vi "Game of colours.vi"() -> ()   [LabVIEW 2018]
uses:
  TypeDefs/State.ctl
  TypeDefs/Application Data.ctl
panel:
  in  "Type the sequence shown":T1
  out "Score":i32
  out "sequence to memorize":u32(colorbox) caption="Sequence to memorize"
  # "The game of colours"
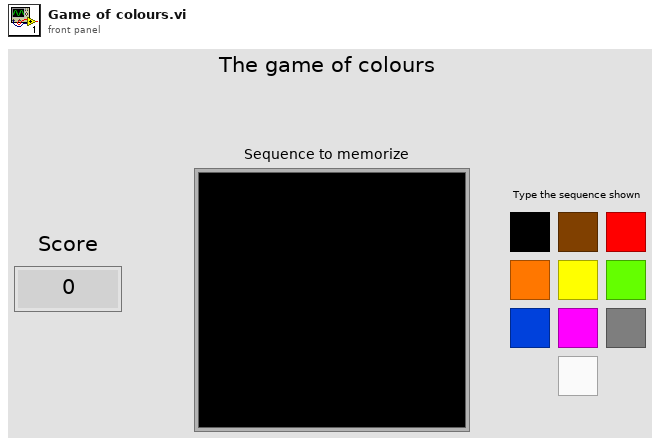
[diagram p1: front panel]
types:
  T1 = cluster{"0":bool, "7":bool, "8":bool, "9":bool, "4":bool, "5":bool, "6":bool, "1":bool, "2":bool, "3":bool}
  T2 = typedef "Application Data.ctl" = cluster{"Sequence":i32[], "Available Colours":u32[], "Wait Time(ms)":u32, "No. Keys Pressed":i32, "Last Key":i16, "Tally":i32}
  T3 = typedef "State.ctl" = enum16{"Initialize", "Add New Colour", "Show Sequence", "Wait for Event", "Check Key Press", "Success", "Failure", "Exit"}
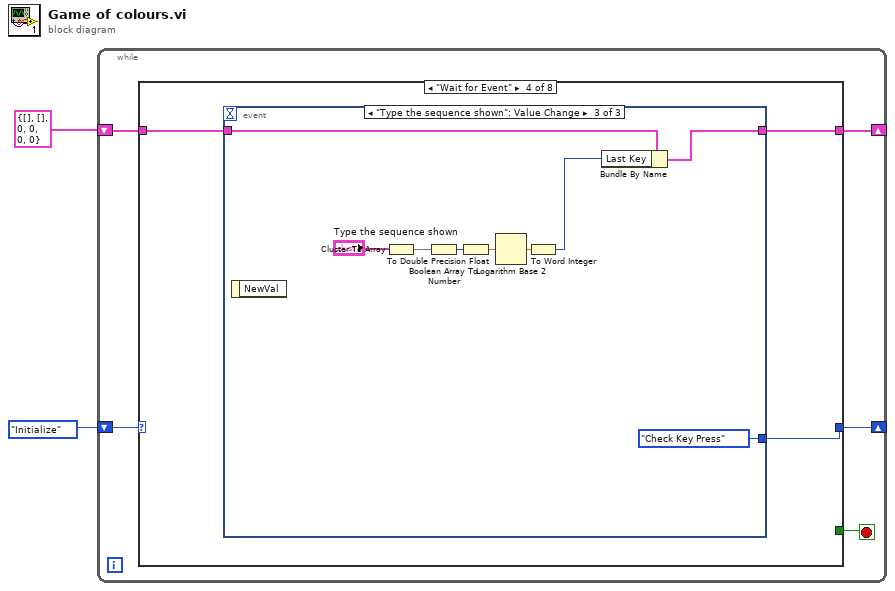
[diagram p0: block diagram]
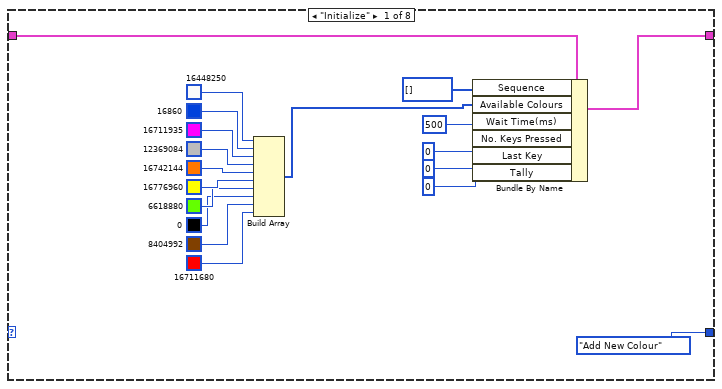
[diagram p2: hidden frame]
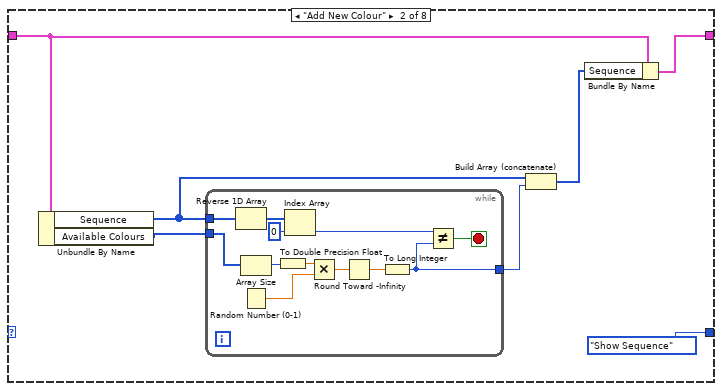
[diagram p3: hidden frame]
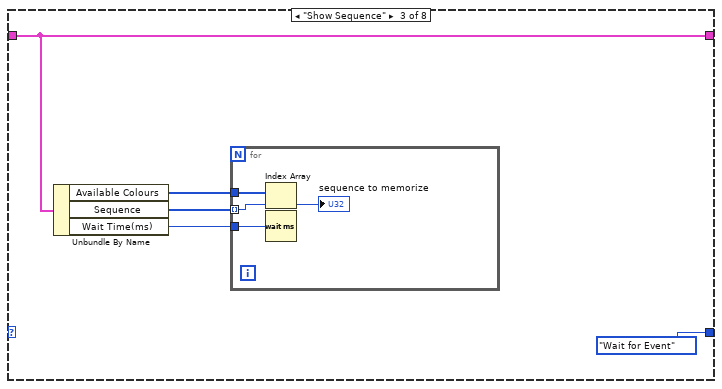
[diagram p4: hidden frame]
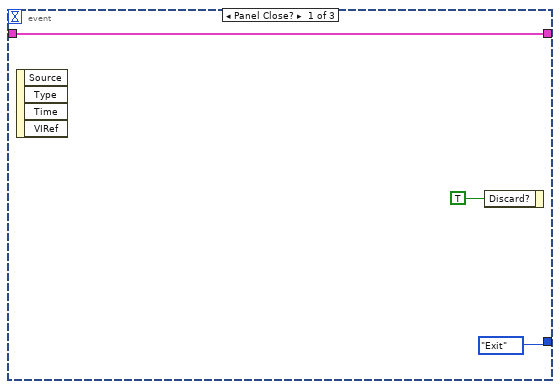
[diagram p5: hidden frame]
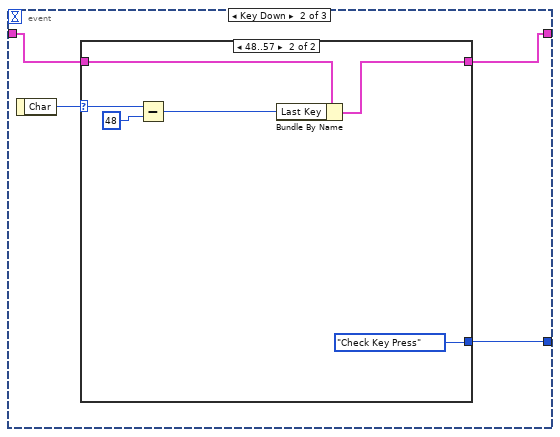
[diagram p6: hidden frame]
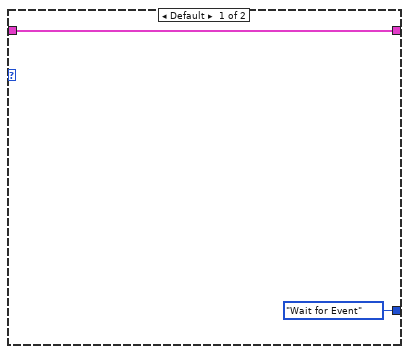
[diagram p7: hidden frame]
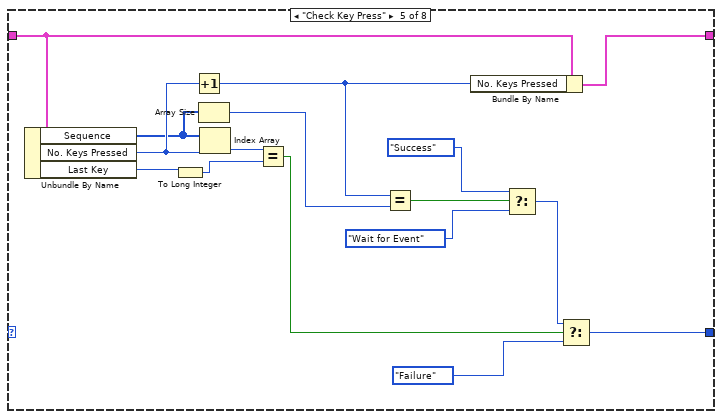
[diagram p8: hidden frame]
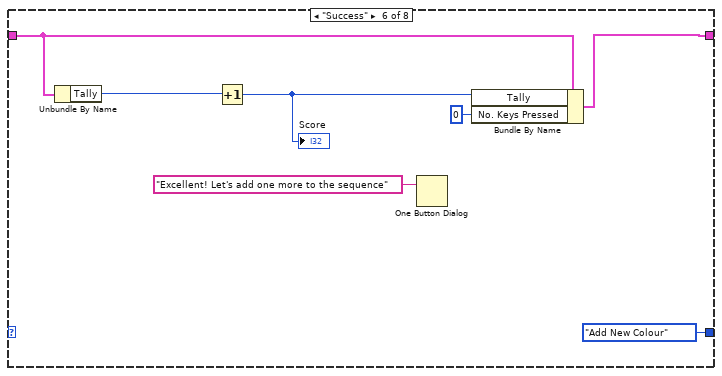
[diagram p9: hidden frame]
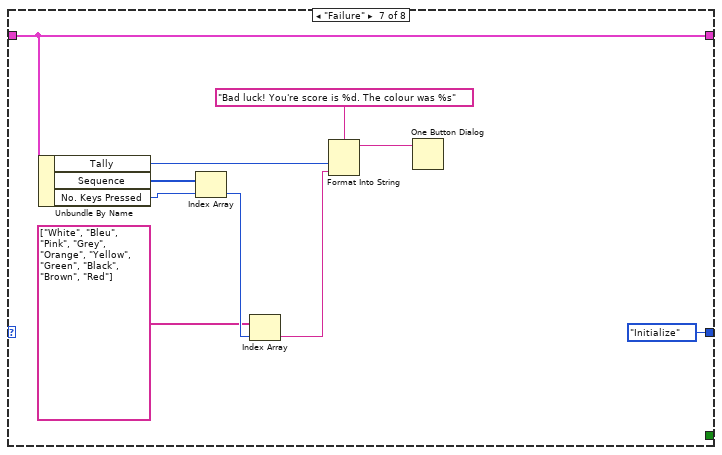
[diagram p10: hidden frame]
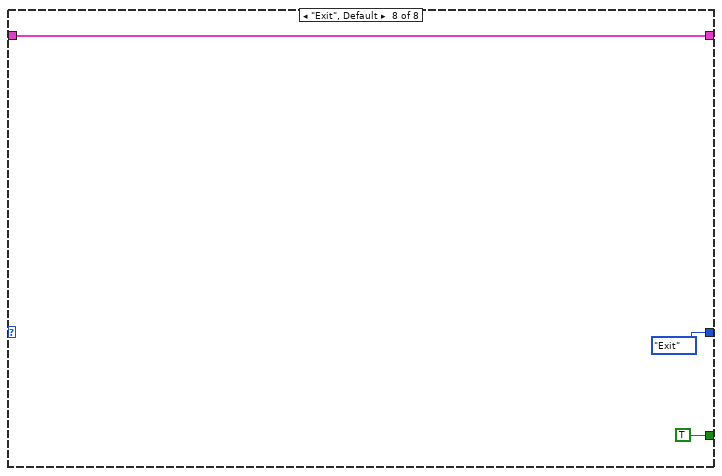
[diagram p11: hidden frame]
diagram:
  n1 = while {
    shift-right: [w4] -> _
    shift-left: T2 {"Sequence"=[], "Available Colours"=[], "Wait Time(ms)"=0, "No. Keys Pressed"=0, "Last Key"=0, "Tally"=0} -> [w5]
    shift-right: [w3] -> _
    shift-left: State."Initialize" -> [w7]
    stop <- w6 stop-if-true
    n2 = case shown="\"Wait for Event\"" w7 {
      tunnel: [_ _ _ _ _ _ _ TRUE] -> w6
      tunnel: [w21 w32 w47 w56 w92 w102 w112 w116] -> w4
      tunnel: w5 -> [w22 w33 w47 w57 w93 w103 w112 w116]
      tunnel: [State."Add New Colour" State."Show Sequence" State."Wait for Event" w55 w86 State."Add New Colour" State."Initialize" State."Exit"] -> w3
      frame "Initialize" {
        n3 = Build Array(u32 16448250 ("Color Box"), u32 16860 ("Color Box"), u32 16711935 ("Color Box"), u32 12369084 ("Color Box"), u32 16742144 ("Color Box"), u32 16776960 ("Color Box"), u32 6618880 ("Color Box"), u32 0 ("Color Box"), u32 8404992 ("Color Box"), u32 16711680 ("Color Box")) -> (w9:u32[])
        n4 = Bundle By Name(cluster=w22, "Sequence"=i32[] [], "Available Colours"=w9, "Wait Time(ms)"=u32 500, "No. Keys Pressed"=0, "Last Key"=i16 0, "Tally"=0) -> (w21:T2)
      }
      frame "Add New Colour" {
        n5 = Unbundle By Name(w33) -> ("Sequence"=w29:i32[], "Available Colours"=w31:u32[])
        n6 = while {
          tunnel: w29 -> [w45]
          tunnel: w31 -> [w42]
          tunnel: [w34] -> w28
          stop <- w35 stop-if-true
          n7 = Reverse 1D Array(array=w45) -> (reversed array=w44:i32[])
          n8 = Array Size(array=w42) -> (size(s)=w40:i32)
          n9 = Random Number (0-1)() -> (number: 0 to 1=w43:dbl)
          n10 = To Double Precision Float(number=w40) -> (double precision float=w39:dbl)
          n11 = Index Array(array=w44, index=0) -> (element=w36:i32)
          n12 = Multiply(x=w39, y=w43) -> (x*y=w41:dbl)
          n13 = Round Toward -Infinity(1:w41) -> (0:w37:dbl)
          n14 = To Long Integer(number=w37) -> (32bit integer=w34:i32)
          n15 = Not Equal?(x=w36, y=w34) -> (x != y?=w35:bool)
        }
        n16 = Build Array (concatenate)(w29, w28) -> (w30:i32[])
        n17 = Bundle By Name(cluster=w33, "Sequence"=w30) -> (w32:T2)
      }
      frame "Show Sequence" {
        n18 = Unbundle By Name(w47) -> ("Available Colours"=w49:u32[], "Sequence"=w50:i32[], "Wait Time(ms)"=w48:u32)
        n19 = for {
          tunnel: w50 -> [w53] mode=indexing
          tunnel: w49 -> [w54]
          tunnel: w48 -> [w51]
          n20 = Index Array(array=w54, index=w53) -> (element=→"sequence to memorize":u32)
          n21 = Wait (ms)(milliseconds to wait=w51) -> ()  [unwired: 1 out]
        }
      }
      frame "Wait for Event" {
        n22 = event shown="[2] \"Type the sequence shown\": Value Change" {
          selector: _ -> [_ _ _]
          dyn-events: _ -> [_ _ _]
          timeout: _ -> [_ _ _]
          tunnel: w57 -> [w59 w63 w76]
          tunnel: [w59 w62 w77] -> w56
          tunnel: [State."Exit" w61 State."Check Key Press"] -> w55
          event Panel Close? {
            n23 = event-data() -> ()  [unwired: 1 in, 4 out]
            n24 = event-data("Discard?"=TRUE) -> ()  [unwired: 1 in, 1 out]
          }
          event Key Down {
            n25 = event-data() -> ("Char"=w64:i16)  [unwired: 1 in]
            n26 = case shown="48..57" w64 {
              selector: w64 -> [_ w69]
              tunnel: w63 -> [w66 w72]
              tunnel: [w66 w71] -> w62
              tunnel: [State."Wait for Event" State."Check Key Press"] -> w61
              frame Default {
              }
              frame 48..57 {
                n27 = Subtract(x=w69, y=i16 48) -> (x-y=w68:i16)
                n28 = Bundle By Name(cluster=w72, "Last Key"=w68) -> (w71:T2)
              }
            }
          }
          event "Type the sequence shown": Value Change {
            n29 = event-data() -> ()  [unwired: 1 in, 1 out]
            n30 = Cluster To Array(cluster="Type the sequence shown") -> (array=w80:bool[])
            n31 = Boolean Array To Number(Boolean array=w80) -> (number=w79:u32)
            n32 = To Double Precision Float(number=w79) -> (double precision float=w78:dbl)
            n33 = Logarithm Base 2(1:w78) -> (0:w75:dbl)
            n34 = To Word Integer(number=w75) -> (16bit integer=w74:i16)
            n35 = Bundle By Name(cluster=w76, "Last Key"=w74) -> (w77:T2)
          }
        }
      }
      frame "Check Key Press" {
        n36 = Unbundle By Name(w93) -> ("Sequence"=w84:i32[], "No. Keys Pressed"=w94:i32, "Last Key"=w96:i16)
        n37 = To Long Integer(number=w96) -> (32bit integer=w95:i32)
        n38 = Increment(x=w94) -> (x+1=w82:i32)
        n39 = Array Size(array=w84) -> (size(s)=w83:i32)
        n40 = Index Array(array=w84, index=w94) -> (element=w97:i32)
        n41 = Equal?(x=w97, y=w95) -> (x = y?=w90:bool)
        n42 = Equal?(x=w82, y=w83) -> (x = y?=w85:bool)
        n43 = Bundle By Name(cluster=w93, "No. Keys Pressed"=w82) -> (w92:T2)
        n44 = Select(t=State."Success", s=w85, f=State."Wait for Event") -> (s? t:f=w87:T3)
        n45 = Select(t=w87, s=w90, f=State."Failure") -> (s? t:f=w86:T3)
      }
      frame "Success" {
        n46 = Unbundle By Name(w103) -> ("Tally"=w99:i32)
        n47 = Increment(x=w99) -> (x+1=w98:i32)
        "Score" <- w98
        n48 = One Button Dialog(message="Excellent! Let's add one more to the sequence") -> ()  [unwired: 1 in, 1 out]
        n49 = Bundle By Name(cluster=w103, "Tally"=w98, "No. Keys Pressed"=0) -> (w102:T2)
      }
      frame "Failure" {
        n50 = Unbundle By Name(w112) -> ("Tally"=w111:i32, "Sequence"=w110:i32[], "No. Keys Pressed"=w109:i32)
        n51 = Index Array(array=w110, index=w109) -> (element=w108:i32)
        n52 = Index Array(array=string[] ["White", "Bleu", "Pink", "Grey", "Orange", "Yellow", "Green", "Black", "Brown", "Red"], index=w108) -> (element=w106:string)
        n53 = Format Into String(format string="Bad luck! You're score is %d. The colour was %s" ("message"), w111, w106) -> (resulting string=w114:string)  [unwired: 2 in, 1 out]
        n54 = One Button Dialog(message=w114) -> ()  [unwired: 1 in, 1 out]
      }
      frame "Exit", Default {
      }
    }
  }
